vi "2-Greater Than Ten.vi"() -> ()   [LabVIEW 2014]
panel:
  in  "Stop Button":bool
  out "Iterations":i32
  out "Greater Than 10":bool
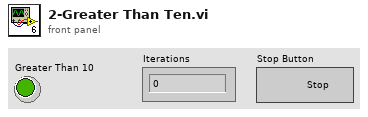
[diagram p1: front panel]
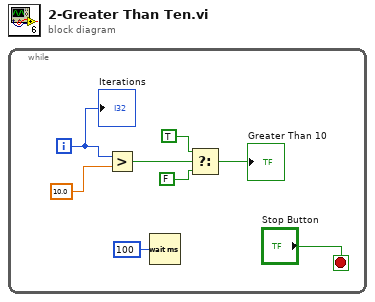
[diagram p0: block diagram]
diagram:
  n1 = while {
    i -> [w6]
    stop <- "Stop Button" stop-if-true
    n2 = Greater?(x=w6, y=10.0) -> (0:w7:bool)
    n3 = Wait (ms)(milliseconds to wait=u32 100) -> ()  [unwired: 1 out]
    n4 = Select(t=TRUE, s=w7, f=FALSE) -> (s? t:f=→"Greater Than 10":bool)
    "Iterations" <- w6
  }
